vi "Autonomous Independent.vi"() -> ()   [LabVIEW 2012]
doc: "This VI is called when autonomous begins, and will automatically be terminated when autonomous ends. You can carry out timed or sensor driven robot movement independently without needing to return to the caller."
uses:
  <vilib>/Rock Robotics/WPI/RobotDrive/WPI_RobotDriveDevRef.ctl
  <vilib>/Rock Robotics/WPI/MotorControl/WPI_MotorControlDeviceRef.ctl
  <vilib>/Rock Robotics/SystemInterfaces/Typedef/FPGA_TypedefDigitalModule.ctl
  <vilib>/Rock Robotics/SystemInterfaces/DIO/FPGA_DIOPWMChannel.ctl
  <vilib>/Rock Robotics/WPI/PWM/WPI_PWMDeadband.ctl
  <vilib>/Rock Robotics/WPI/CAN/Jaguar/SubVIs/WPI_CANJaguar_ControlMode.ctl
  <vilib>/Rock Robotics/WPI/PWM/WPI_PWMTransform_ConPane.ctl
  Robot Global Data.vi
  <vilib>/Rock Robotics/WPI/RobotDrive/WPI_RobotDriveGetSetRefNum.vi
  <vilib>/Rock Robotics/WPI/Joystick/WPI_JoystickGetSetRefNum.vi
  <vilib>/Rock Robotics/WPI/RobotDrive/WPI_RobotDriveArcadeDrive_Standard(NoSaturation).vi
panel:
  in  "RobotDriveDevRef 3":T1={"DevStatus"={"status"=FALSE, "code"=0, "source"=""}, "Motors[]"=[], "Square Inputs"=FALSE, "Max Output"=1.0, "Isochronous"=FALSE}
  in  "RobotDriveDevRef 2":T1={"DevStatus"={"status"=FALSE, "code"=0, "source"=""}, "Motors[]"=[], "Square Inputs"=FALSE, "Max Output"=1.0, "Isochronous"=FALSE}
  in  "RobotDriveDevRef":T1={"DevStatus"={"status"=FALSE, "code"=0, "source"=""}, "Motors[]"=[], "Square Inputs"=FALSE, "Max Output"=1.0, "Isochronous"=FALSE}
  out "Stop":bool
  in  "Array":dbl[][](array[numeric])
  out "Distance":bool
  out "Shoot":bool
  out "Rotate":bool
  out "millisecond timer value":u32
  out "Current Movement, for debugging":T9 {"Y Joystick Value" scale=1.0..-1.0; "X Joystick Value" scale=-1.0..1.0}
  in  "Array of robot movements":T10(array[cluster]) {"Y Joystick Value" scale=1.0..-1.0; "X Joystick Value" scale=-1.0..1.0}
  # "Be sure to right-click and choose Data Operations>>Make Current Value default if you want to save the array values with the VI"
  # "Shoot"
  # "Stop"
  # "Time"
  # "Rotate"
  # "Distance"
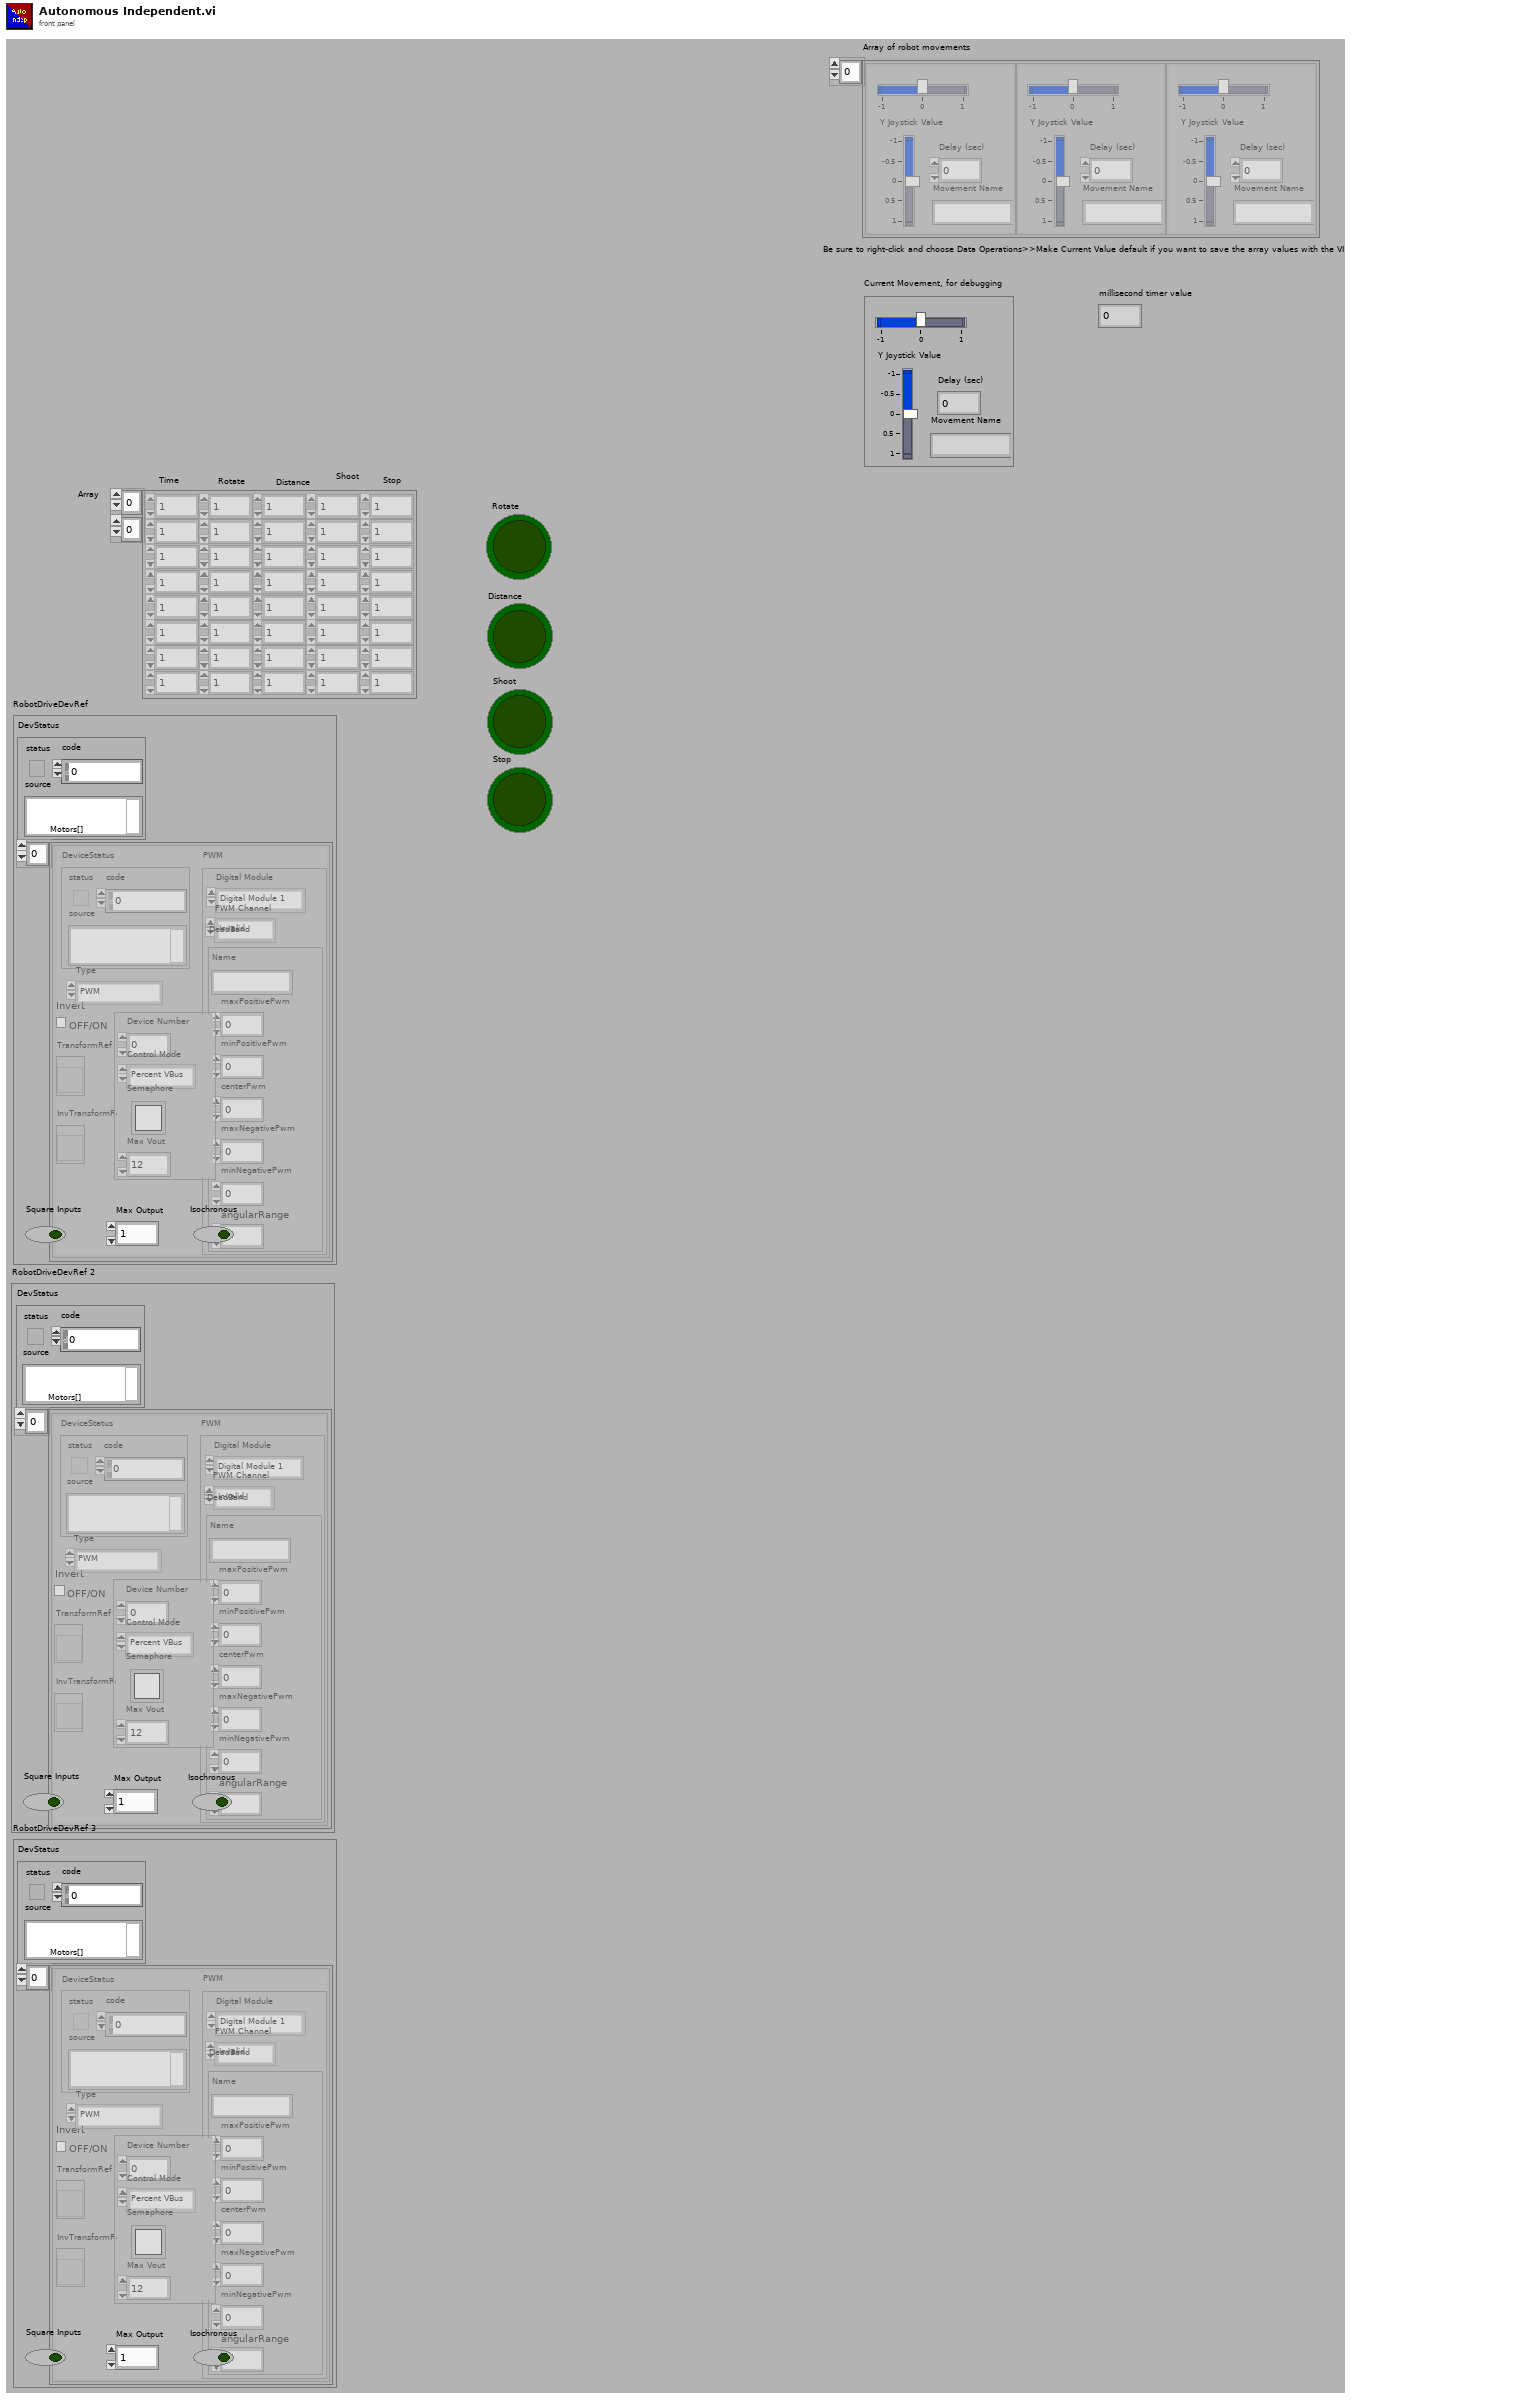
[diagram p1: front panel]
types:
  T1 = typedef "WPI_RobotDriveDevRef.ctl" = cluster{"DevStatus":errorcluster, "Motors[]":T2[], "Square Inputs":bool, "Max Output":dbl, "Isochronous":bool}
  T2 = typedef "WPI_MotorControlDeviceRef.ctl" = cluster{"DeviceStatus":errorcluster, "Type":enum16{"PWM", "CAN"}, "PWM":cluster{"Digital Module":T3, "PWM Channel":T4, "DeadBand":T5}, "CAN":cluster{"Device Number":u8, "Control Mode":T6, "Semaphore":T7, "Max Vout":dbl}, "Invert":bool, "TransformRef":T8, "InvTransformRef":T8}
  T3 = typedef "FPGA_TypedefDigitalModule.ctl" = enum16{"Digital Module 1", "Digital Module 2"}
  T4 = typedef "FPGA_DIOPWMChannel.ctl" = enum8{"PWM 1", "PWM 2", "PWM 3", "PWM 4", "PWM 5", "PWM 6", "PWM 7", "PWM 8", "PWM 9", "PWM 10", "Invalid"}
  T5 = typedef "WPI_PWMDeadband.ctl" = cluster{"Name":string, "maxPositivePwm":i32, "minPositivePwm":i32, "centerPwm":i32, "maxNegativePwm":i32, "minNegativePwm":i32, "angularRange":u16}
  T6 = typedef "WPI_CANJaguar_ControlMode.ctl" = enum8{"Percent VBus", "Current", "Speed", "Position", "Voltage"}
  T7 = typedef "Semaphore RefNum" = refnum<k1>
  T8 = typedef "WPI_PWMTransform_ConPane.ctl" = refnum<vi>
  T9 = cluster{"X Joystick Value":dbl, "Y Joystick Value":dbl, "Delay (sec)":dbl, "Movement Name":string}
  T10 = cluster{"X Joystick Value":dbl, "Y Joystick Value":dbl, "Delay (sec)":dbl, "Movement Name":string}[]
  T11 = typedef "WPI_JoystickDevRef.ctl" = cluster{"Device":T12}
  T12 = typedef "WPI_JoystickDeviceEnum.ctl" = enum16{"USB 1", "USB 2", "USB 3", "USB 4", "Kinect 1", "Kinect 2"}
  T13 = cluster{"axis 1 (x)":dbl, "axis 2 (y)":dbl, "axis 3 (throttle)":dbl, "axis 4":dbl, "axis 5":dbl, "axis 6":dbl}
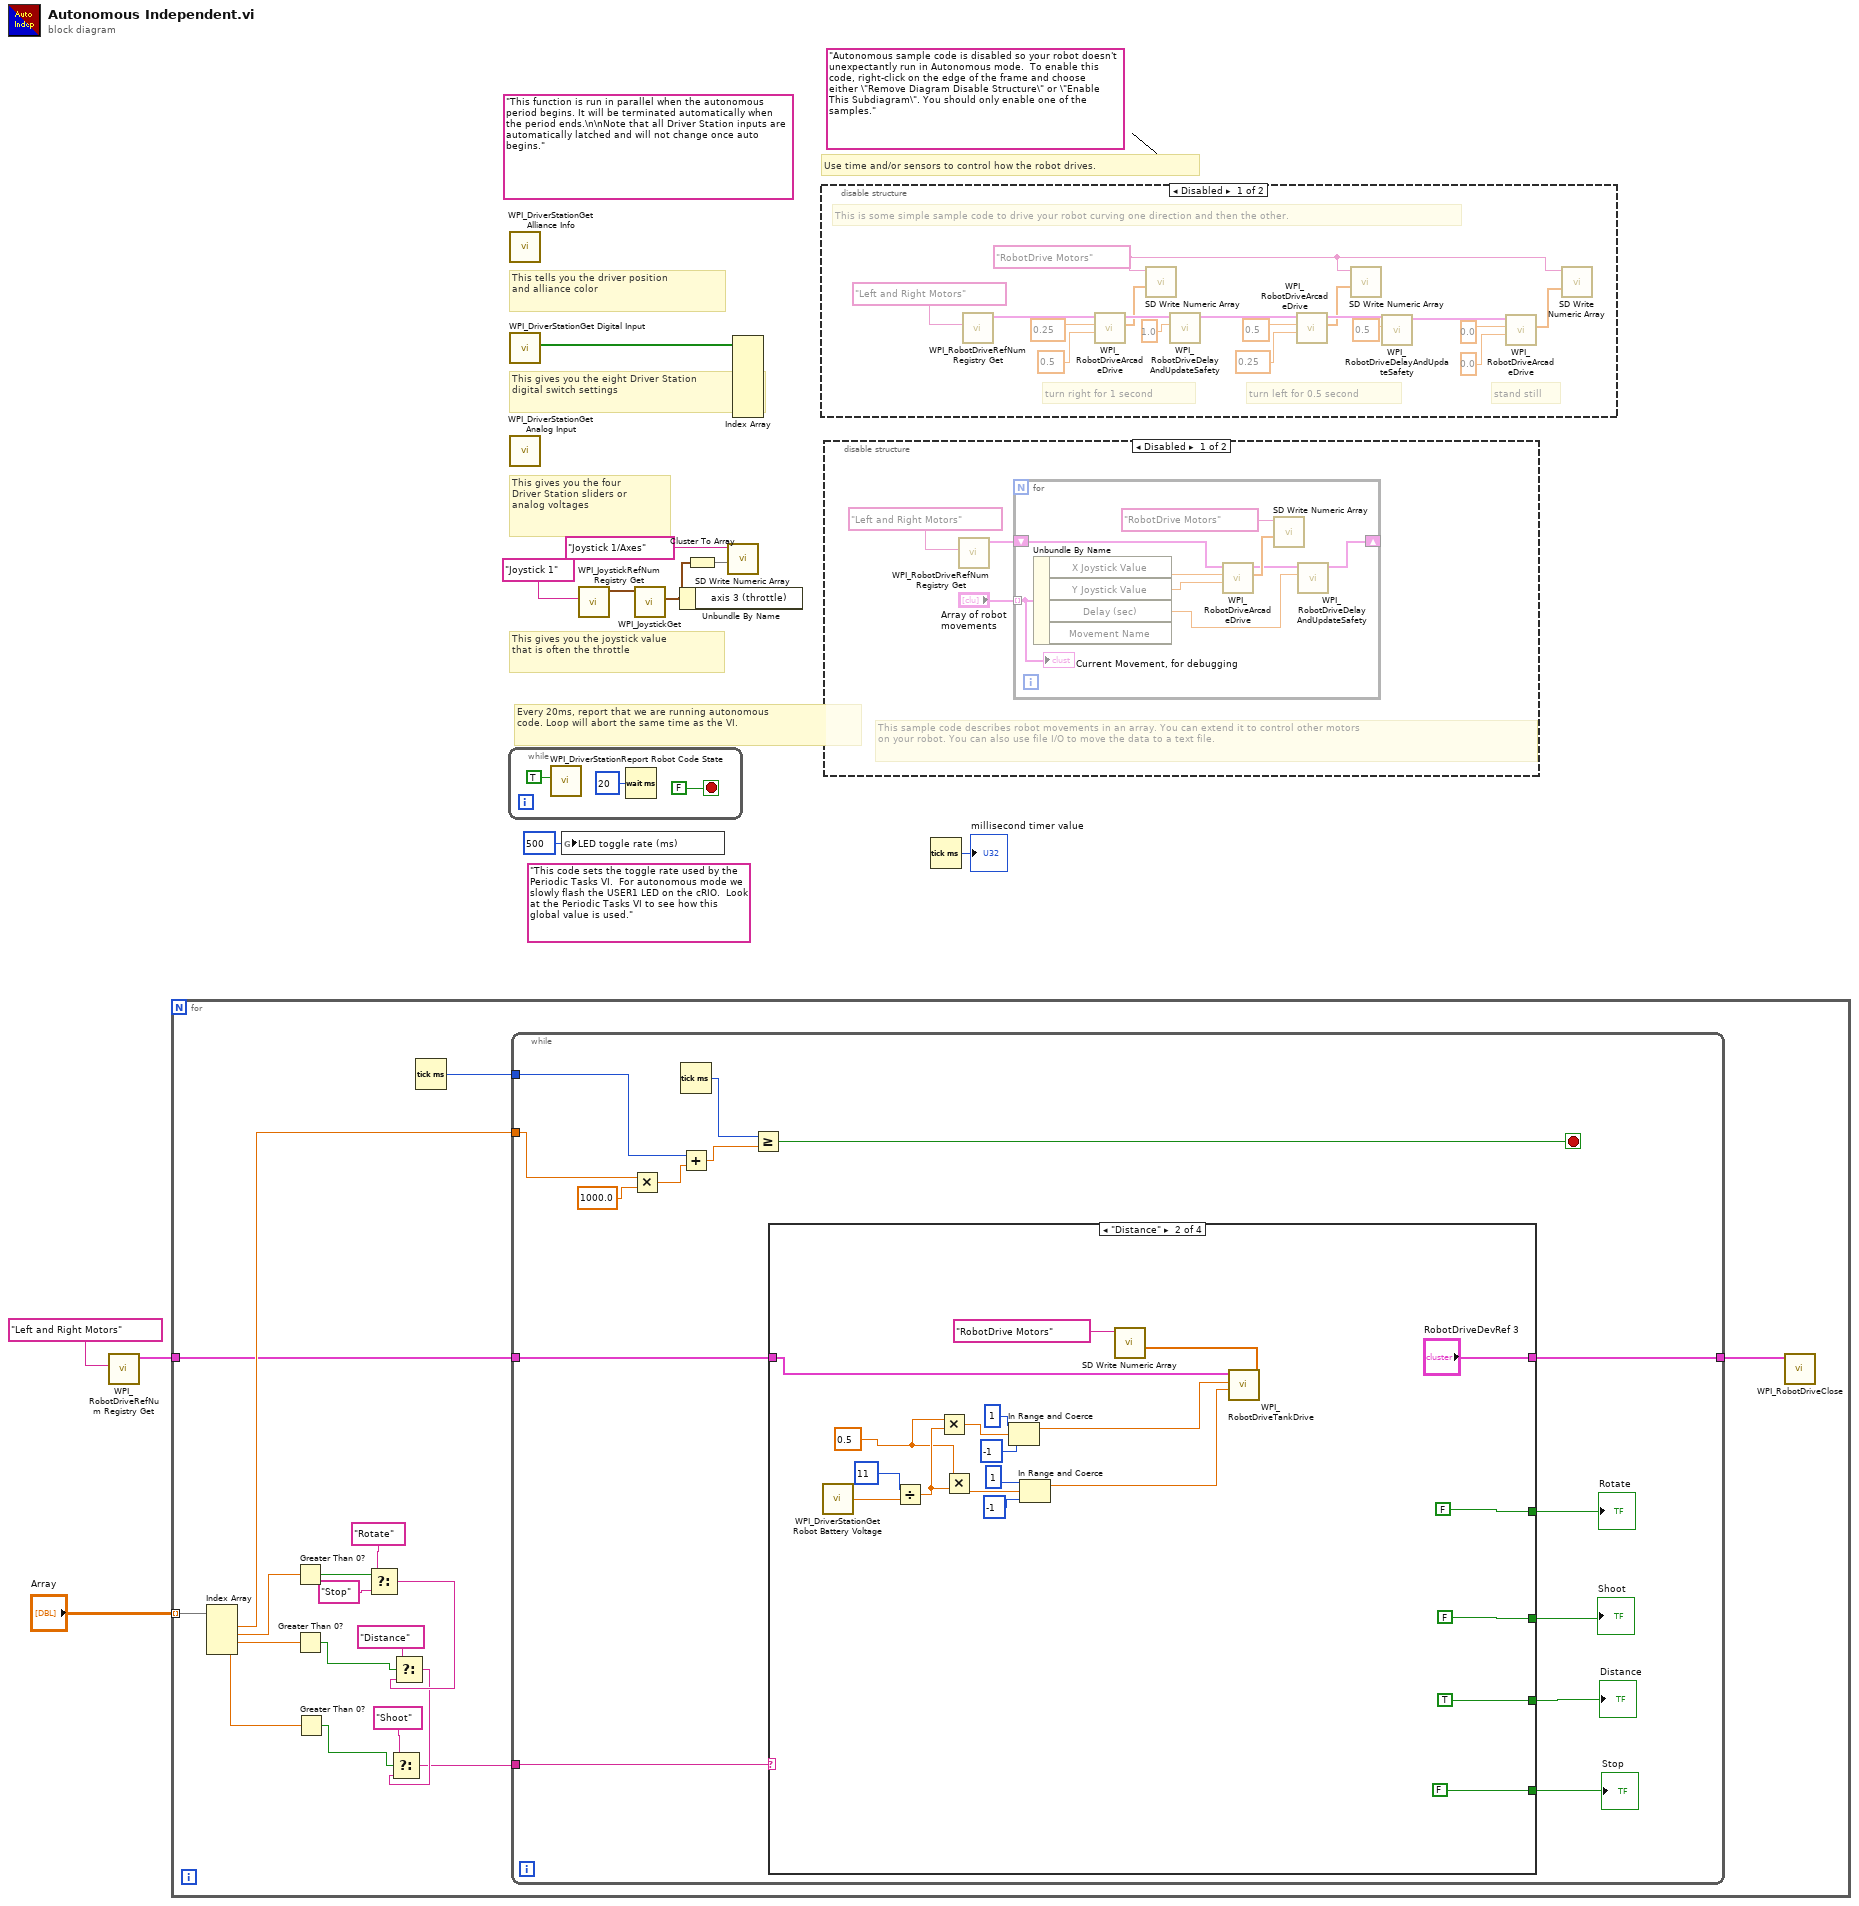
[diagram p0: block diagram]
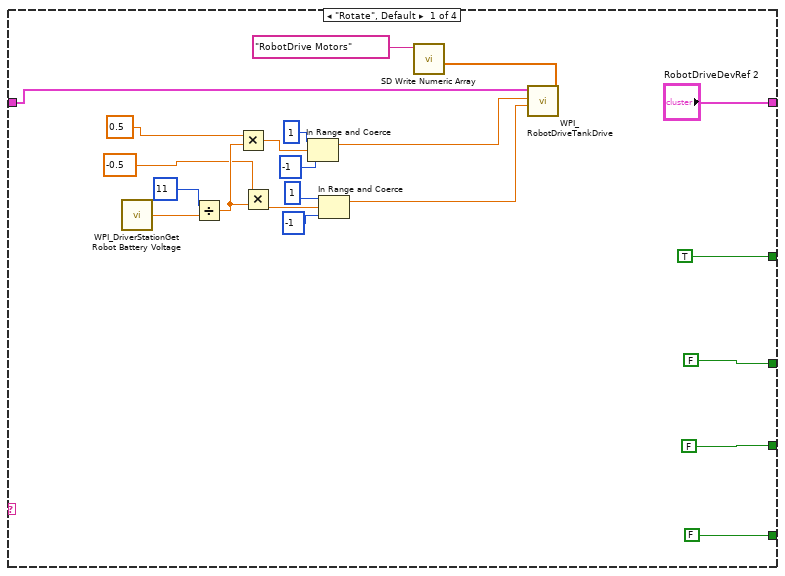
[diagram p2: hidden frame]
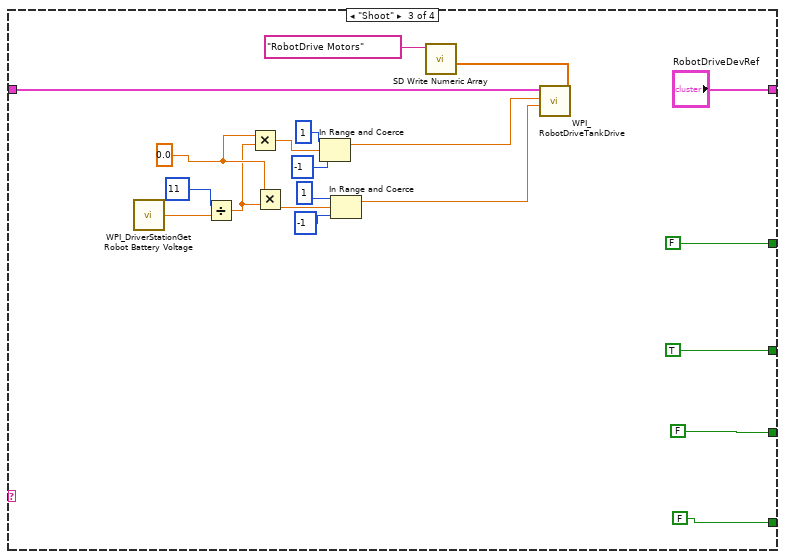
[diagram p3: hidden frame]
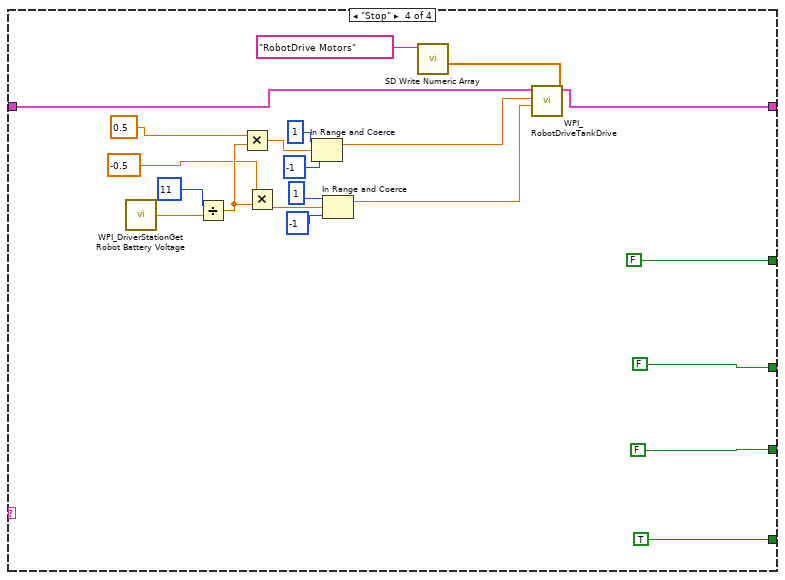
[diagram p4: hidden frame]
diagram:
  (unwired) "This code sets the toggle rate used by the Periodic Tasks VI.  For autonomous mode we slowly flash the USER1 LED on the cRIO.  Look at the Periodic Tasks VI to see how this global value is used."
  (unwired) "Autonomous sample code is disabled so your robot doesn't unexpectantly run in Autonomous mode.  To enable this code, right-click on the edge of the frame and choose either \"Remove Diagram Disable Structure\" or \"Enable This Subdiagram\". You should only enable one of the samples."
  (unwired) "This function is run in parallel when the autonomous period begins. It will be terminated automatically when the period ends.\n\nNote that all Driver Station inputs are automatically latched and will not change once auto begins."
  # "Every 20ms, report that we are running autonomous\ncode. Loop will abort the same time as the VI."
  # "This gives you the joystick value\nthat is often the throttle"
  # "Use time and/or sensors to control how the robot drives."
  # "This tells you the driver position\nand alliance color"
  # "This gives you the eight Driver Station\ndigital switch settings"
  # "This gives you the four\nDriver Station sliders or\nanalog voltages"
  n1 = call <vilib>:"WPI_RobotDriveRefNum Registry Get.vi"("refnum name"="Left and Right Motors") -> ("RobotDriveDevRef"=w1:T1)  [unwired: 1 in, 9 out]
  n2 = for {
    tunnel: "Array" -> [w29] mode=indexing
    tunnel: w1 -> [w13]
    n3 = Index Array(array=w29) -> (element #1=w16:dbl, element #2=w28:dbl, element #3=w27:dbl, element #4=w26:dbl)  [unwired: 4 in]
    n4 = Greater Than 0?(x=w28) -> (x > 0?=w25:bool)
    n5 = Greater Than 0?(x=w27) -> (x > 0?=w21:bool)
    n6 = Greater Than 0?(x=w26) -> (x > 0?=w19:bool)
    n7 = Select(t="Rotate", s=w25, f="Stop") -> (s? t:f=w18:string)
    n8 = Select(t="Distance", s=w21, f=w18) -> (s? t:f=w17:string)
    n9 = Select(t="Shoot", s=w19, f=w17) -> (s? t:f=w14:string)
    n10 = Tick Count (ms)() -> (millisecond timer value=w15:u32)
    n11 = while {
      tunnel: w16 -> [w41]
      tunnel: w15 -> [w39]
      tunnel: w14 -> [w36]
      tunnel: w13 -> [w32]
      tunnel: [w31] -> w12
      stop <- w37 stop-if-true
      n12 = Multiply(x=w41, y=1000.0) -> (x*y=w40:dbl)
      n13 = Tick Count (ms)() -> (millisecond timer value=w42:u32)
      n14 = Add(x=w39, y=w40) -> (x+y=w38:dbl)
      n15 = Greater Or Equal?(x=w42, y=w38) -> (x >= y?=w37:bool)
      n16 = case shown="\"Distance\"" w36 {
        tunnel: [FALSE ("Rotate") TRUE ("Distance") FALSE ("Rotate") FALSE ("Rotate")] -> w35
        tunnel: [FALSE ("Rotate") FALSE ("Rotate") TRUE ("Shoot") FALSE ("Rotate")] -> w34
        tunnel: [TRUE ("Rotate") FALSE ("Rotate") FALSE ("Rotate") FALSE ("Rotate")] -> w33
        tunnel: w32 -> [w46 w67 w87 w106]
        tunnel: ["RobotDriveDevRef 2" "RobotDriveDevRef 3" "RobotDriveDevRef" w105] -> w31
        tunnel: [FALSE ("Rotate") FALSE ("Rotate") FALSE ("Rotate") TRUE ("Rotate")] -> w30
        frame "Rotate", Default {
          n17 = call <vilib>:"WPI_DriverStationGet Robot Battery Voltage.vi"() -> ("robot battery voltage"=w59:dbl)  [unwired: 14 in, 1 out]
          n18 = Divide(x=11, y=w59) -> (x/y=w57:dbl)
          n19 = Multiply(x=0.5, y=w57) -> (x*y=w54:dbl)
          n20 = Multiply(x=-0.5, y=w57) -> (x*y=w53:dbl)
          n21 = In Range and Coerce(upper limit=1, x=w54, lower limit=-1) -> (coerced(x)=w50:dbl)  [unwired: 1 out]
          n22 = In Range and Coerce(upper limit=1, x=w53, lower limit=-1) -> (coerced(x)=w49:dbl)  [unwired: 1 out]
          n23 = call <vilib>:"WPI_RobotDriveTankDrive.vi"("Right axis value"=w49, "Left axis value"=w50, "RobotDriveDevRef"=w46) -> ("Motor Values"=w60:dbl[])  [unwired: 6 in, 2 out]
          n24 = call <vilib>:"SD Write Numeric Array.vi"("Numeric Array"=w60, "Name"="RobotDrive Motors") -> ()  [unwired: 8 in, 2 out]
        }
        frame "Distance" {
          w68 = 0.5 ("x")
          n25 = call <vilib>:"WPI_DriverStationGet Robot Battery Voltage.vi"() -> ("robot battery voltage"=w79:dbl)  [unwired: 14 in, 1 out]
          n26 = Divide(x=11, y=w79) -> (x/y=w77:dbl)
          n27 = Multiply(x=w68, y=w77) -> (x*y=w74:dbl)
          n28 = Multiply(x=w68, y=w77) -> (x*y=w73:dbl)
          n29 = In Range and Coerce(upper limit=1, x=w74, lower limit=-1) -> (coerced(x)=w70:dbl)  [unwired: 1 out]
          n30 = In Range and Coerce(upper limit=1, x=w73, lower limit=-1) -> (coerced(x)=w69:dbl)  [unwired: 1 out]
          n31 = call <vilib>:"WPI_RobotDriveTankDrive.vi"("Right axis value"=w69, "Left axis value"=w70, "RobotDriveDevRef"=w67) -> ("Motor Values"=w80:dbl[])  [unwired: 6 in, 2 out]
          n32 = call <vilib>:"SD Write Numeric Array.vi"("Numeric Array"=w80, "Name"="RobotDrive Motors") -> ()  [unwired: 8 in, 2 out]
        }
        frame "Shoot" {
          w101 = 0.0 ("x")
          n33 = call <vilib>:"WPI_DriverStationGet Robot Battery Voltage.vi"() -> ("robot battery voltage"=w90:dbl)  [unwired: 14 in, 1 out]
          n34 = Divide(x=11, y=w90) -> (x/y=w92:dbl)
          n35 = Multiply(x=w101, y=w92) -> (x*y=w95:dbl)
          n36 = Multiply(x=w101, y=w92) -> (x*y=w96:dbl)
          n37 = In Range and Coerce(upper limit=1, x=w95, lower limit=-1) -> (coerced(x)=w99:dbl)  [unwired: 1 out]
          n38 = In Range and Coerce(upper limit=1, x=w96, lower limit=-1) -> (coerced(x)=w100:dbl)  [unwired: 1 out]
          n39 = call <vilib>:"WPI_RobotDriveTankDrive.vi"("Right axis value"=w100, "Left axis value"=w99, "RobotDriveDevRef"=w87) -> ("Motor Values"=w89:dbl[])  [unwired: 6 in, 2 out]
          n40 = call <vilib>:"SD Write Numeric Array.vi"("Numeric Array"=w89, "Name"="RobotDrive Motors") -> ()  [unwired: 8 in, 2 out]
        }
        frame "Stop" {
          n41 = call <vilib>:"WPI_DriverStationGet Robot Battery Voltage.vi"() -> ("robot battery voltage"=w119:dbl)  [unwired: 14 in, 1 out]
          n42 = Divide(x=11, y=w119) -> (x/y=w117:dbl)
          n43 = Multiply(x=0.5, y=w117) -> (x*y=w114:dbl)
          n44 = Multiply(x=-0.5, y=w117) -> (x*y=w113:dbl)
          n45 = In Range and Coerce(upper limit=1, x=w114, lower limit=-1) -> (coerced(x)=w110:dbl)  [unwired: 1 out]
          n46 = In Range and Coerce(upper limit=1, x=w113, lower limit=-1) -> (coerced(x)=w109:dbl)  [unwired: 1 out]
          n47 = call <vilib>:"WPI_RobotDriveTankDrive.vi"("Right axis value"=w109, "Left axis value"=w110, "RobotDriveDevRef"=w106) -> ("Motor Values"=w120:dbl[], "RobotDriveDevRef"=w105:T1)  [unwired: 6 in, 1 out]
          n48 = call <vilib>:"SD Write Numeric Array.vi"("Numeric Array"=w120, "Name"="RobotDrive Motors") -> ()  [unwired: 8 in, 2 out]
        }
      }
      "Distance" <- w35
      "Shoot" <- w34
      "Rotate" <- w33
      "Stop" <- w30
    }
    n49 = call <vilib>:"WPI_RobotDriveClose.vi"("RobotDriveDevRef"=w12) -> ()  [unwired: 10 in, 1 out]
  }
  n50 = while {
    stop <- FALSE stop-if-true
    n51 = call <vilib>:"WPI_DriverStationReport Robot Code State.vi"("Autonomous"=TRUE) -> ()  [unwired: 10 in, 1 out]
    n52 = Wait (ms)(milliseconds to wait=u32 20) -> ()  [unwired: 1 out]
  }
  n53 = call <vilib>:"WPI_DriverStationGet Alliance Info.vi"() -> ()  [unwired: 12 out]
  n54 = call <vilib>:"WPI_DriverStationGet Digital Input.vi"() -> ("Driver Station Digital Input (1-8)"=w11:bool[])  [unwired: 11 out]
  n55 = call <vilib>:"WPI_DriverStationGet Analog Input.vi"() -> ()  [unwired: 12 out]
  n56 = global write "Robot Global Data.vi" "LED toggle rate (ms)"(u32 500 ("LED ms toggle rate")) -> ()
  n57 = call <vilib>:"WPI_JoystickRefNum Registry Get.vi"("refnum name"="Joystick 1") -> ("JoystickDevRef"=w9:T11)  [unwired: 1 in, 9 out]
  n58 = call <vilib>:"WPI_JoystickGet.vi"("JoystickDevRef"=w9) -> ("Axes"=w6:T13)  [unwired: 1 in, 5 out]
  n59 = Unbundle By Name(w6) -> ()  [unwired: 1 out]
  n60 = Cluster To Array(cluster=w6) -> (array=w7:dbl[])
  n61 = call <vilib>:"SD Write Numeric Array.vi"("Numeric Array"=w7, "Name"="Joystick 1/Axes") -> ()  [unwired: 8 in, 2 out]
  n62 = Index Array(array=w11) -> ()  [unwired: 8 in, 8 out]
  n63 = disable-structure shown="Disabled" {
    frame Disabled {
      w129 = "RobotDrive Motors" ("Name")
      # "This is some simple sample code to drive your robot curving one direction and then the other."
      # "stand still"
      # "turn left for 0.5 second"
      # "turn right for 1 second"
      n64 = call <vilib>:"WPI_RobotDriveRefNum Registry Get.vi"("refnum name"="Left and Right Motors") -> ("RobotDriveDevRef"=w133:T1)  [unwired: 1 in, 9 out]
      n65 = call-poly <vilib>:"WPI_RobotDriveArcadeDrive.vi"("Y axis value"=0.5 ("X axis value"), "X axis value"=0.25, "RobotDriveDevRef"=w133) -> ("Motor Values"=w132:dbl[], "RobotDriveDevRef"=w140:T1)  [unwired: 1 in, 6 out]
      n66 = call <vilib>:"SD Write Numeric Array.vi"("Numeric Array"=w132, "Name"=w129) -> ()  [unwired: 8 in, 2 out]
      n67 = call <vilib>:"WPI_RobotDriveDelayAndUpdateSafety.vi"("Delay (s)"=1.0, "RobotDriveDevRef"=w140) -> ("RobotDriveDevRef 2"=w139:T1)  [unwired: 8 in, 1 out]
      n68 = call-poly <vilib>:"WPI_RobotDriveArcadeDrive.vi"("Y axis value"=0.25 ("X axis value"), "X axis value"=0.5, "RobotDriveDevRef"=w139) -> ("Motor Values"=w131:dbl[], "RobotDriveDevRef"=w138:T1)  [unwired: 1 in, 6 out]
      n69 = call <vilib>:"SD Write Numeric Array.vi"("Numeric Array"=w131, "Name"=w129) -> ()  [unwired: 8 in, 2 out]
      n70 = call <vilib>:"WPI_RobotDriveDelayAndUpdateSafety.vi"("Delay (s)"=0.5, "RobotDriveDevRef"=w138) -> ("RobotDriveDevRef 2"=w137:T1)  [unwired: 8 in, 1 out]
      n71 = call-poly <vilib>:"WPI_RobotDriveArcadeDrive.vi"("Y axis value"=0.0 ("X axis value"), "X axis value"=0.0, "RobotDriveDevRef"=w137) -> ("Motor Values"=w130:dbl[])  [unwired: 1 in, 7 out]
      n72 = call <vilib>:"SD Write Numeric Array.vi"("Numeric Array"=w130, "Name"=w129) -> ()  [unwired: 8 in, 2 out]
    }
    frame Enabled {
    }
  }
  n73 = disable-structure shown="Disabled" {
    frame Disabled {
      # "This sample code describes robot movements in an array. You can extend it to control other motors\non your robot. You can also use file I/O to move the data to a text file."
      n74 = call <vilib>:"WPI_RobotDriveRefNum Registry Get.vi"("refnum name"="Left and Right Motors") -> ("RobotDriveDevRef"=w148:T1)  [unwired: 1 in, 9 out]
      n75 = for {
        shift-right: [w154] -> _
        shift-left: w148 -> [w155]
        tunnel: "Array of robot movements" -> [w150] mode=indexing
        n76 = Unbundle By Name(w150) -> ("X Joystick Value"=w153:dbl, "Y Joystick Value"=w152:dbl, "Delay (sec)"=w151:dbl)  [unwired: 1 out]
        n77 = call-poly <vilib>:"WPI_RobotDriveArcadeDrive.vi"("Y axis value"=w152, "X axis value"=w153, "RobotDriveDevRef"=w155) -> ("Motor Values"=w157:dbl[], "RobotDriveDevRef"=w156:T1)  [unwired: 1 in, 6 out]
        n78 = call <vilib>:"SD Write Numeric Array.vi"("Numeric Array"=w157, "Name"="RobotDrive Motors") -> ()  [unwired: 8 in, 2 out]
        n79 = call <vilib>:"WPI_RobotDriveDelayAndUpdateSafety.vi"("Delay (s)"=w151, "RobotDriveDevRef"=w156) -> ("RobotDriveDevRef 2"=w154:T1)  [unwired: 8 in, 1 out]
        "Current Movement, for debugging" <- w150
      }
    }
    frame Enabled {
    }
  }
  n80 = Tick Count (ms)() -> (millisecond timer value=→"millisecond timer value":u32)
